vi "myDAQ_DMM.vi"() -> ()   [LabVIEW 2023]
panel:
  out "Most Recent Measurement":dbl
  out "Plot":dynamicdata(graph)
  in  "stop":bool
  in  "Measurement Type":enum16{"Voltage", "Current", "Resistance"}(ring)
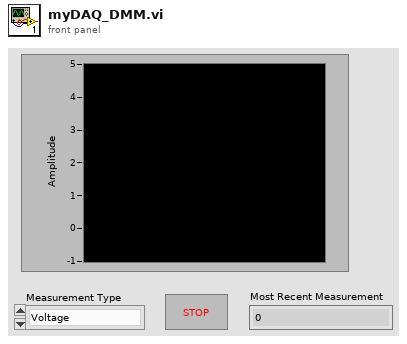
[diagram p1: front panel]
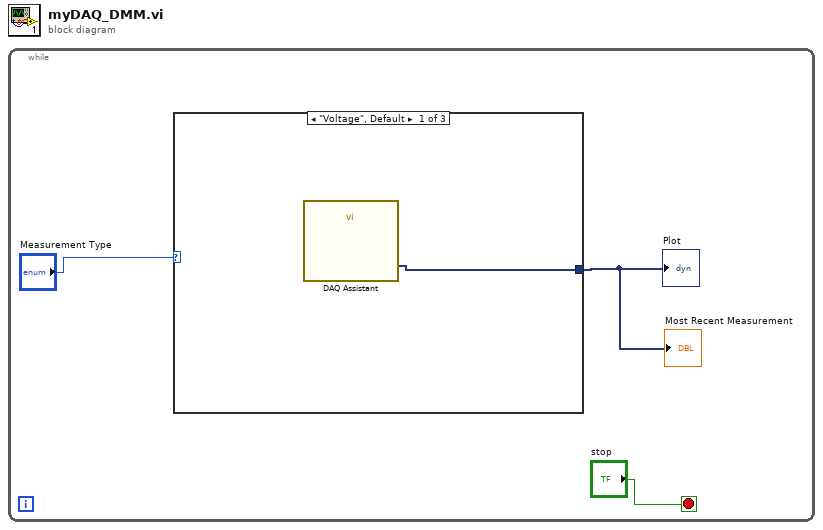
[diagram p0: block diagram]
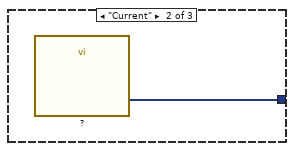
[diagram p2: hidden frame]
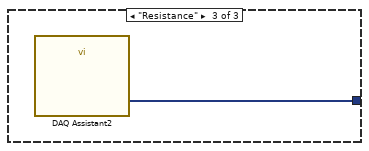
[diagram p3: hidden frame]
diagram:
  n1 = while {
    stop <- "stop" stop-if-true
    n2 = case shown="\"Voltage\", Default" "Measurement Type" {
      tunnel: [w4 w5 w6] -> w1
      frame "Voltage", Default {
        n3 = call "DAQ Assistant"() -> ("data"=w4:dynamicdata)  [unwired: 17 in, 2 out]
      }
      frame "Current" {
        n4 = call "?"() -> ("data"=w5:dynamicdata)  [unwired: 17 in, 2 out]
      }
      frame "Resistance" {
        n5 = call "DAQ Assistant2"() -> ("data"=w6:dynamicdata)  [unwired: 17 in, 2 out]
      }
    }
    "Plot" <- w1
    "Most Recent Measurement" <- w1
  }
